vi "Reaffirm_ADAM_Outputs.vi"(3 "Channel Description":T1[](array[typedef]) {"Duty" format="%.0b"; "D" format="%#_5g"; "C" format="%#_5g"; "B" format="%#_5g"; "A" format="%#_5g"}, 4 "Active Ch Indicies":i32[](array[numeric]), 5 "Current Channel Values":dbl[](array[numeric]) format="%.2f") -> (1 "Scan Comments":string[](array[string]))   [LabVIEW 2013]
uses:
  ADAM Client/Sub VIs/ADAM Controls/Ch_description_ADAM.ctl
  ADAM Client/Sub VIs/ADAM Controls/Module_type_ADAM.ctl
  ADAM Client/Sub VIs/ADAM Controls/Function_ADAM.ctl
  ADAM Client/Sub VIs/ADAM Controls/Channel_State.ctl
  ADAM Client/Sub VIs/ADAM Controls/Calib_type_ADAM.ctl
  ADAM Client/Sub VIs/ADAM Controls/Address.ctl
  ADAM_Global.vi
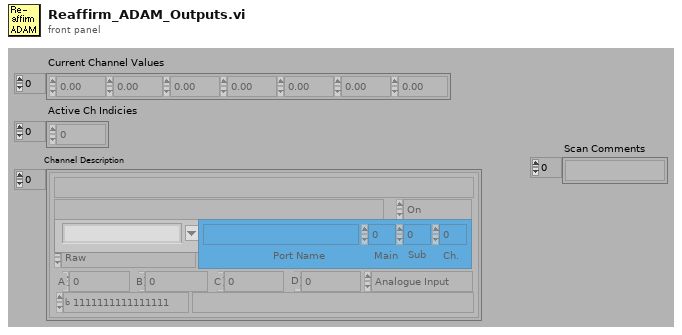
[diagram p1: front panel]
types:
  T1 = typedef "Ch_description_ADAM.ctl" = cluster{"Ch Name":string, "Type":T2, "Function":T3, "Ch State":T4, "Calibration type":T5, "A":dbl, "B":dbl, "C":dbl, "D":dbl, "Comments":string, "Address":T6, "String":string, "Duty":u16}
  T2 = typedef "Module_type_ADAM.ctl" = string
  T3 = typedef "Function_ADAM.ctl" = enum16{"Analogue Input", "Digital Input", "Event counter", "Event rate", "Analogue Output", "Digital Output", "Relay Output"}
  T4 = typedef "Channel_State.ctl" = enum16{"On", "Off", "Always On", "Always Off"}
  T5 = typedef "Calib_type_ADAM.ctl" = enum16{"Raw", "Bx + A", "Cx^2 + Bx + A", "Dx^3 + Cx^2 + Bx + A", "In Band", "Hi-Tec Q", "Hi-Tec M_dot", "Text"}
  T6 = typedef "Address.ctl" = cluster{"Main":i32, "Ch.":i32, "Sub":i32, "Port Name":string}
  T7 = typedef "Server_Control.ctl" = cluster{"Channel Name to control":string, "Channel sharing":enum16{"Channel Unshared", "Channel Shared by Rig", "Channel Shared by Group"}, "Default Value":dbl, "Client Array":string[], "Time Stamp":timestamp, "Do Not Reset":bool}
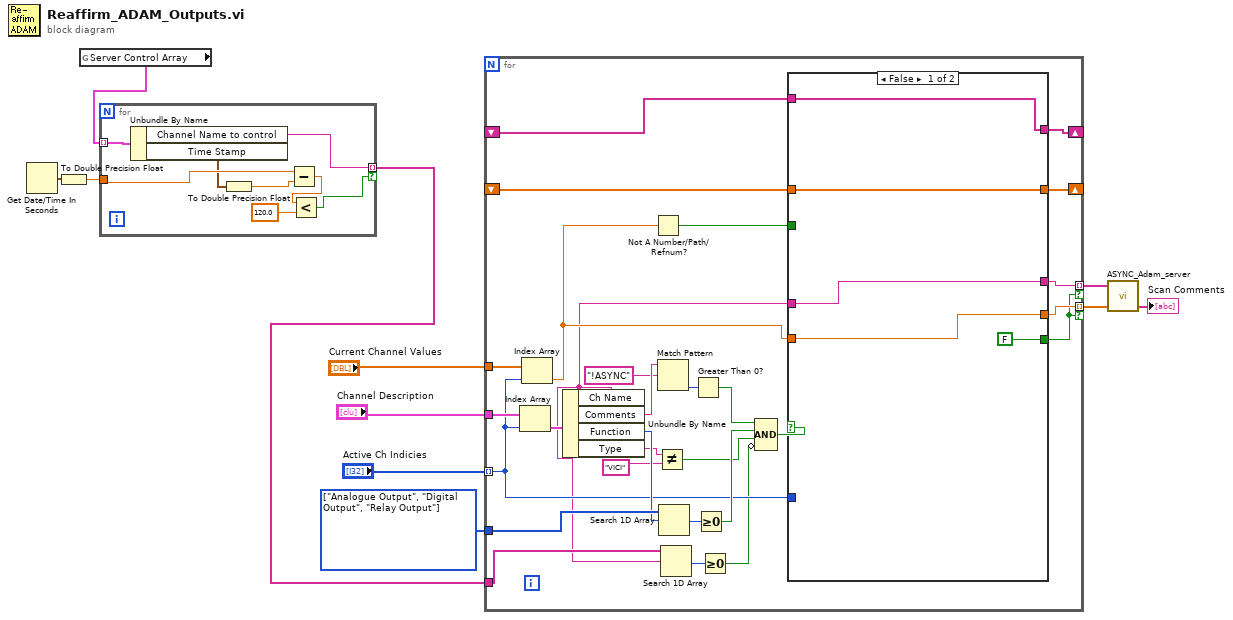
[diagram p0: block diagram]
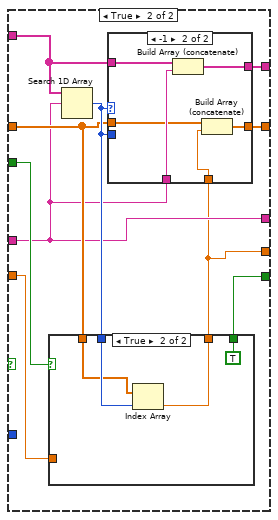
[diagram p2: hidden frame]
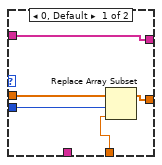
[diagram p3: hidden frame]
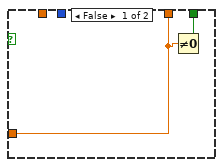
[diagram p4: hidden frame]
diagram:
  w9 = T3[] [enum."Analogue Output", enum."Digital Output", enum."Relay Output"] items=["Analogue Input", "Digital Input", "Event counter", "Event rate", "Analogue Output", "Digital Output", "Relay Output"]
  n1 = Get Date/Time In Seconds() -> (seconds since 1Jan1904=w5:timestamp)
  n2 = To Double Precision Float(number=w5) -> (double precision float=w4:dbl)
  n3 = global read "ADAM_Global.vi" "Server Control Array"() -> (w6:T7[])
  n4 = for {
    tunnel: w6 -> [w19] mode=indexing
    tunnel: w4 -> [w18]
    tunnel: [w13] -> w1 mode=indexing if=w12
    n5 = Unbundle By Name(w19) -> ("Channel Name to control"=w13:string, "Time Stamp"=w17:timestamp)
    n6 = To Double Precision Float(number=w17) -> (double precision float=w16:dbl)
    n7 = Subtract(x=w18, y=w16) -> (x-y=w15:dbl)
    n8 = Less?(x=w15, y=120.0) -> (x < y?=w12:bool)
  }
  n9 = for {
    tunnel: "Channel Description" -> [w38]
    tunnel: "Active Ch Indicies" -> [w36] mode=indexing
    tunnel: w9 -> [w47]
    tunnel: "Current Channel Values" -> [w37]
    shift-right: [w31] -> _
    shift-left: _ -> [w32]
    shift-right: [w29] -> _
    shift-left: _ -> [w30]
    tunnel: w1 -> [w26]
    tunnel: [w22] -> w3 mode=indexing if=w20
    tunnel: [w21] -> w2 mode=indexing if=w20
    n10 = Index Array(array=w38, index=w36) -> (element=w48:T1)
    n11 = Index Array(array=w37, index=w36) -> (element=w28:dbl)
    n12 = Unbundle By Name(w48) -> ("Ch Name"=w25:string, "Comments"=w45:string, "Function"=w46:T3, "Type"=w35:T2)
    n13 = Not A Number/Path/Refnum?(number/path/refnum=w28) -> (NaN/Path/Refnum?=w27:bool)
    n14 = Not Equal?(x=w35, y=T2 "VICI" ("Type")) -> (x != y?=w33:bool)
    n15 = Match Pattern(string=w45, regular expression="!ASYNC") -> (offset past match=w43:i32)  [unwired: 4 out]
    n16 = Search 1D Array(1D array=w47, element=w46) -> (index of element=w42:i32)  [unwired: 1 out]
    n17 = Search 1D Array(1D array=w26, element=w25) -> (index of element=w24:i32)  [unwired: 1 out]
    n18 = Greater Than 0?(x=w43) -> (x > 0?=w40:bool)
    n19 = Greater Or Equal To 0?(x=w42) -> (x >= 0?=w41:bool)
    n20 = Greater Or Equal To 0?(x=w24) -> (x >= 0?=w23:bool)
    n21 = Compound Arithmetic op=AND(w40, w41, w33, invert w23) -> (w39:bool)
    n22 = case shown="False" w39 {
      tunnel: w36 -> [_ _]
      tunnel: [w50 w55] -> w22
      tunnel: w25 -> [w51 w56]
      tunnel: [w51 w56] -> w21
      tunnel: w28 -> [w50 w60]
      tunnel: w32 -> [w53 w63]
      tunnel: [w53 w62] -> w31
      tunnel: w30 -> [w52 w58]
      tunnel: [w52 w61] -> w29
      tunnel: w27 -> [_ w57]
      tunnel: [FALSE w54] -> w20
      frame False {
      }
      frame True {
        n23 = Search 1D Array(1D array=w63, element=w56) -> (index of element=w59:i32)  [unwired: 1 out]
        n24 = case shown="True" w57 {
          tunnel: [w76 w78] -> w55
          tunnel: w60 -> [w76 _]
          tunnel: w59 -> [_ w80]
          tunnel: w58 -> [_ w79]
          tunnel: [w75 TRUE] -> w54
          frame False {
            n25 = Not Equal To 0?(x=w76) -> (x != 0?=w75:bool)
          }
          frame True {
            n26 = Index Array(array=w79, index=w80) -> (element=w78:dbl)
          }
        }
        n27 = case shown="-1" w59 {
          tunnel: w63 -> [w68 w74]
          tunnel: w56 -> [_ w73]
          tunnel: [w68 w72] -> w62
          tunnel: w59 -> [w67 _]
          tunnel: w58 -> [w66 w71]
          tunnel: [w65 w69] -> w61
          tunnel: w55 -> [w64 w70]
          frame 0, Default {
            n28 = Replace Array Subset(array=w66, new element=w64, index=w67) -> (w65:dbl[])
          }
          frame -1 {
            n29 = Build Array (concatenate)(w74, w73) -> (w72:string[])
            n30 = Build Array (concatenate)(w71, w70) -> (w69:dbl[])
          }
        }
      }
    }
  }
  n31 = call "ASYNC_Adam_server.vi"("Values"=w3, "Channel Names"=w2) -> ("Scan Comments"=→"Scan Comments":string[])  [unwired: 1 in, 2 out]
